vi "Stop Core.vi"(10 "final error code":i32, 11 "MCListbox View in":refnum<class "MCListbox View.lvclass">) -> (3 "MCListbox View out":refnum<class "MCListbox View.lvclass">)   [LabVIEW 2013, in "SET Project Editor.lvlib" / "MCListbox View.lvclass"]
doc: "(<B>Filename</B>: Actor Framework.lvlib:Actor.lvclass:Stop Core.vi)\n\nDefines what the actor does before it stops. Use the <B>final error code</B> input to determine whether the actor shut down in response to an error.\n\nBy default, this method does nothing. A descendant class may override it to define behavior, such as shutting down any processes the actor initiated in its override of the Actor Core method."
uses:
  MCListbox View.lvclass
  UI View/UI View.lvclass
  MCListbox View.lvclass/MCListbox View.ctl
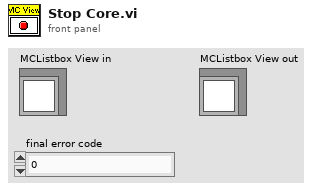
[diagram p1: front panel]
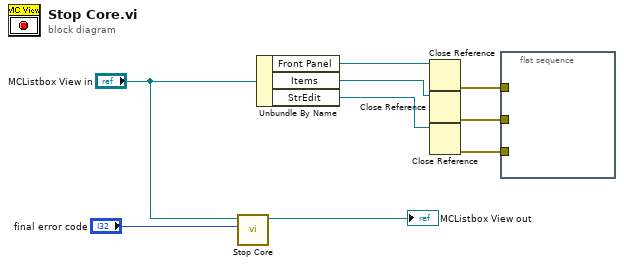
[diagram p0: block diagram]
diagram:
  n1 = call-parent "Stop Core.vi"("final error code"="final error code", "UI Actor in"="MCListbox View in") -> ("UI Actor out"=→"MCListbox View out":refnum<class "MCListbox View.lvclass">)  [unwired: 9 in]
  n2 = Unbundle By Name("MCListbox View in") -> ("Front Panel"=w6:refnum<vi>, "Items"=w5:refnum<vi>, "StrEdit"=w4:refnum<vi>)
  n3 = Close Reference(reference=w6) -> (error out=w1:errorcluster)  [unwired: 1 in]
  n4 = Close Reference(reference=w5) -> (error out=w2:errorcluster)  [unwired: 1 in]
  n5 = Close Reference(reference=w4) -> (error out=w3:errorcluster)  [unwired: 1 in]
  n6 = flat-sequence {
    tunnel: w3 -> [_]
    tunnel: w2 -> [_]
    tunnel: w1 -> [_]
    frame #0 {
    }
  }
